vi "Convert num value to syntax selection.vi"(2 "GCS syntax version":dbl=1.0 min=0.0 max=20.0 step=1.0 format="%.2f") -> (14 "Syntax":T1)   [LabVIEW 2020]
doc: "This VI converts a numerical value to the corresponding GCS syntax version."
uses:
  Communication.llb/Syntax.ctl
panel:
  # "This VI converts a numerical value\nto the corresponding GCS syntax version."
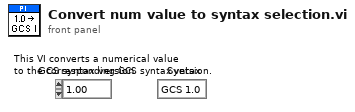
[diagram p1: front panel]
types:
  T1 = typedef "Syntax.ctl" = enum16{"GCS 1.0", "GCS 2.0", "GCS 3.0"}
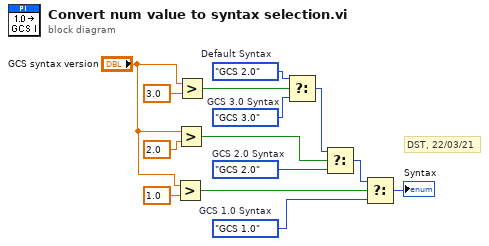
[diagram p0: block diagram]
diagram:
  w4 = Syntax."GCS 2.0"  # Default Syntax
  w6 = Syntax."GCS 3.0"  # GCS 3.0 Syntax
  w9 = Syntax."GCS 2.0"  # GCS 2.0 Syntax
  w12 = Syntax."GCS 1.0"  # GCS 1.0 Syntax
  # "DST, 22/03/21"
  n1 = Greater?(x="GCS syntax version", y=1.0) -> (0:w13:bool)
  n2 = Greater?(x="GCS syntax version", y=2.0) -> (0:w1:bool)
  n3 = Greater?(x="GCS syntax version", y=3.0) -> (0:w8:bool)
  n4 = Select(t=w4, s=w8, f=w6) -> (s? t:f=w5:T1)
  n5 = Select(t=w5, s=w1, f=w9) -> (s? t:f=w10:T1)
  n6 = Select(t=w10, s=w13, f=w12) -> (s? t:f=→"Syntax":T1)
